vi "create pixel 1D array.vi"(8 "error in (no error)":errorcluster, 11 "LineCCD in":refnum<class "LineCCD.lvclass">) -> (0 "error out":errorcluster, 3 "LineCCD out":refnum<class "LineCCD.lvclass">)   [LabVIEW 2012, in "LineCCD.lvclass"]
uses:
  LineCCD.lvclass
  LineCCD.lvclass/LineCCD.ctl
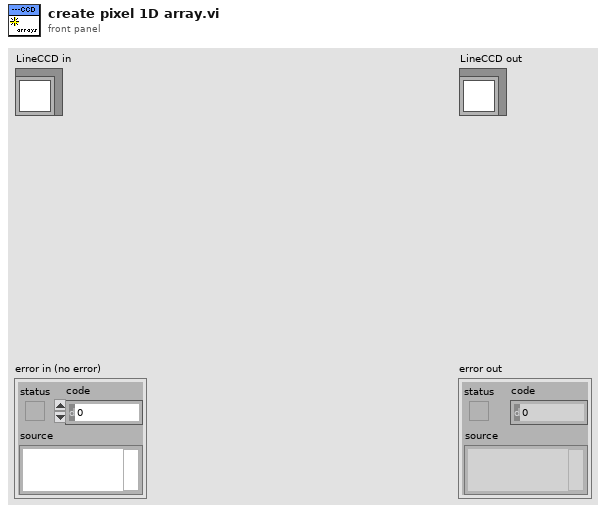
[diagram p1: front panel]
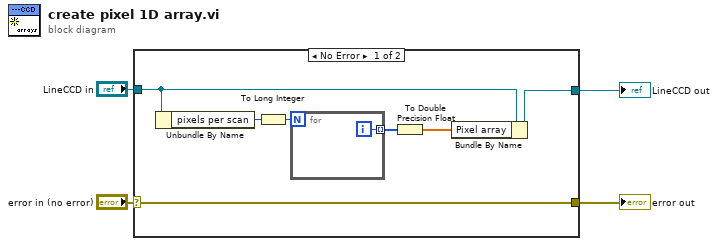
[diagram p0: block diagram]
diagram:
  n1 = case shown="No Error" "error in (no error)" {
    selector: "error in (no error)" -> [w8 w14]
    tunnel: [w8 w14] -> w3
    tunnel: [w6 w13] -> w1
    tunnel: "LineCCD in" -> [w7 w13]
    frame No Error {
      n2 = Unbundle By Name(w7) -> ("pixels per scan"=w10:u32)
      n3 = To Long Integer(number=w10) -> (32bit integer=w11:i32)
      n4 = for {
        N: w11 -> [_]
        tunnel: [w12] -> w9 mode=indexing
        i -> [w12]
      }
      n5 = To Double Precision Float(number=w9) -> (double precision float=w5:dbl[])
      n6 = Bundle By Name(cluster=w7, "Pixel array"=w5) -> (w6:refnum<class "LineCCD.lvclass">)
    }
    frame Error {
    }
  }
  "error out" <- w3
  "LineCCD out" <- w1
